vi "tcp data queue to requested values.vi"(10 "TCP subscriptions info":T1, 11 "Queue in":refnum<queue>) -> (0 "error out":errorcluster, 2 "Array":string[](array[string]), 3 "Queue out":refnum<queue>)   [LabVIEW 2020]
uses:
  TCP subscription info cluster.ctl
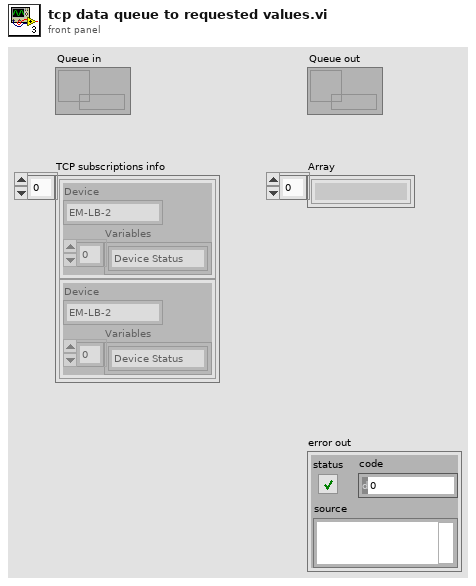
[diagram p1: front panel]
types:
  T1 = typedef "TCP subscription info cluster.ctl" = cluster{"Device":string, "Variables":string[]}[]
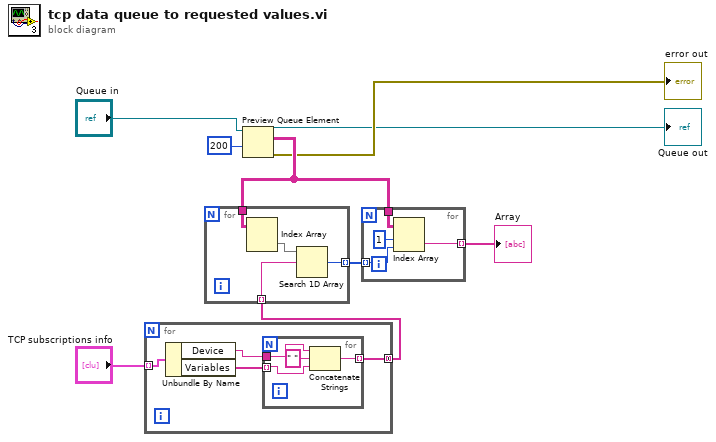
[diagram p0: block diagram]
diagram:
  n1 = for {
    tunnel: "TCP subscriptions info" -> [w13] mode=indexing
    tunnel: [w10] -> w9 mode=concatenating
    n2 = Unbundle By Name(w13) -> ("Device"=w12:string, "Variables"=w11:string[])
    n3 = for {
      tunnel: w12 -> [w16]
      tunnel: w11 -> [w15] mode=indexing
      tunnel: [w14] -> w10 mode=indexing
      n4 = Concatenate Strings(w16, " " ("string"), w15) -> (w14:string)
    }
  }
  n5 = Preview Queue Element(queue="Queue in", timeout in ms (-1)=200) -> (queue out=→"Queue out":refnum<queue>, element=w5:string[][], error out=→"error out":errorcluster)  [unwired: 1 in, 1 out]
  n6 = for {
    tunnel: w5 -> [w21]
    tunnel: w9 -> [w19] mode=indexing
    tunnel: [w18] -> w6 mode=indexing
    n7 = Index Array(array=w21) -> (element=w20:string[])  [unwired: 2 in]
    n8 = Search 1D Array(1D array=w20, element=w19) -> (index of element=w18:i32)  [unwired: 1 in]
  }
  n9 = for {
    tunnel: w5 -> [w25]
    tunnel: w6 -> [w23] mode=indexing
    tunnel: [w22] -> w7 mode=indexing
    n10 = Index Array(array=w25, index (row)=1, index (col)=w23) -> (element=w22:string)
  }
  "Array" <- w7
